vi "Occurance Performance Test.vi"() -> ()   [LabVIEW 2021]
panel:
  out "x-y":dbl format="%#_6p"
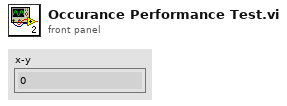
[diagram p1: front panel]
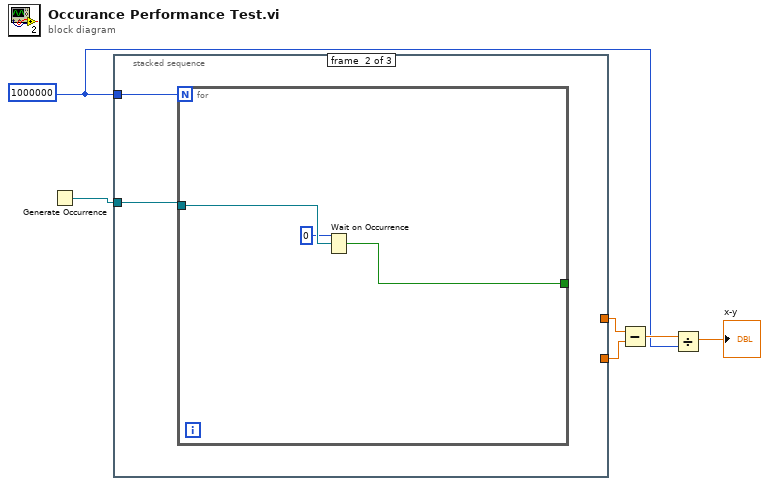
[diagram p0: block diagram]
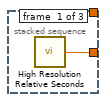
[diagram p2: hidden frame]
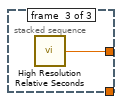
[diagram p3: hidden frame]
diagram:
  w2 = 1000000
  n1 = Generate Occurrence() -> (w1:refnum<k4>)
  n2 = stacked-sequence {
    tunnel: [w7 _ _] -> w6
    tunnel: [_ _ w13] -> w5
    tunnel: w2 -> [_ w9 _]
    tunnel: w1 -> [_ w8 _]
    frame #0 {
      n3 = call <vilib>:"High Resolution Relative Seconds.vi"() -> ("relative seconds"=w7:dbl)
    }
    frame #1 {
      n4 = for {
        N: w9 -> [_]
        tunnel: [w10] -> _
        tunnel: w8 -> [w12]
        n5 = Wait on Occurrence(2:w12, 3:0 ("ms timeout (-1)")) -> (0:w10:bool)  [unwired: 1 in]
      }
    }
    frame #2 {
      n6 = call <vilib>:"High Resolution Relative Seconds.vi"() -> ("relative seconds"=w13:dbl)
    }
  }
  n7 = Subtract(x=w5, y=w6) -> (x-y=w4:dbl)
  n8 = Divide(x=w4, y=w2) -> (x/y=→"x-y":dbl)
